vi "FTW-File-ResolveSymbolicPaths.vi"(0 "Unresolved Path":path, 11 "error in":errorcluster) -> (4 "Resolved Path":path, 15 "error out":errorcluster)   [LabVIEW 2012]
uses:
  Error/FTW-ERR-ThrowError.vi
panel:
  # "Inputs"
  # "Outputs"
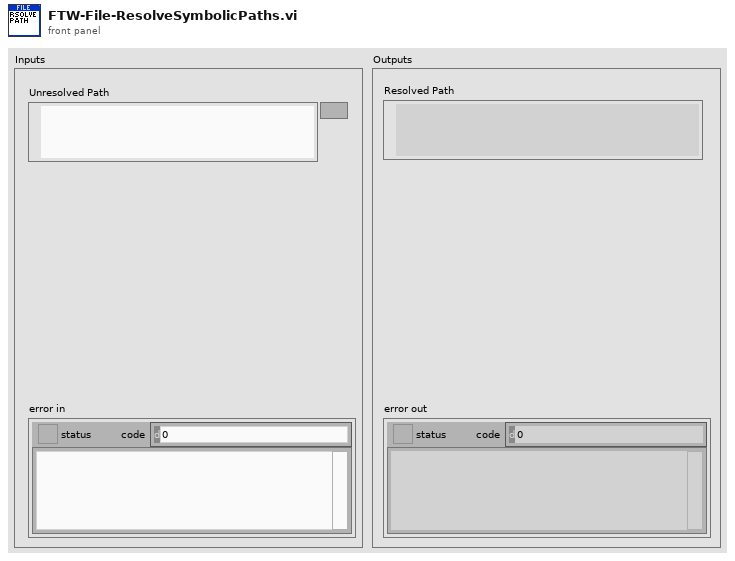
[diagram p1: front panel]
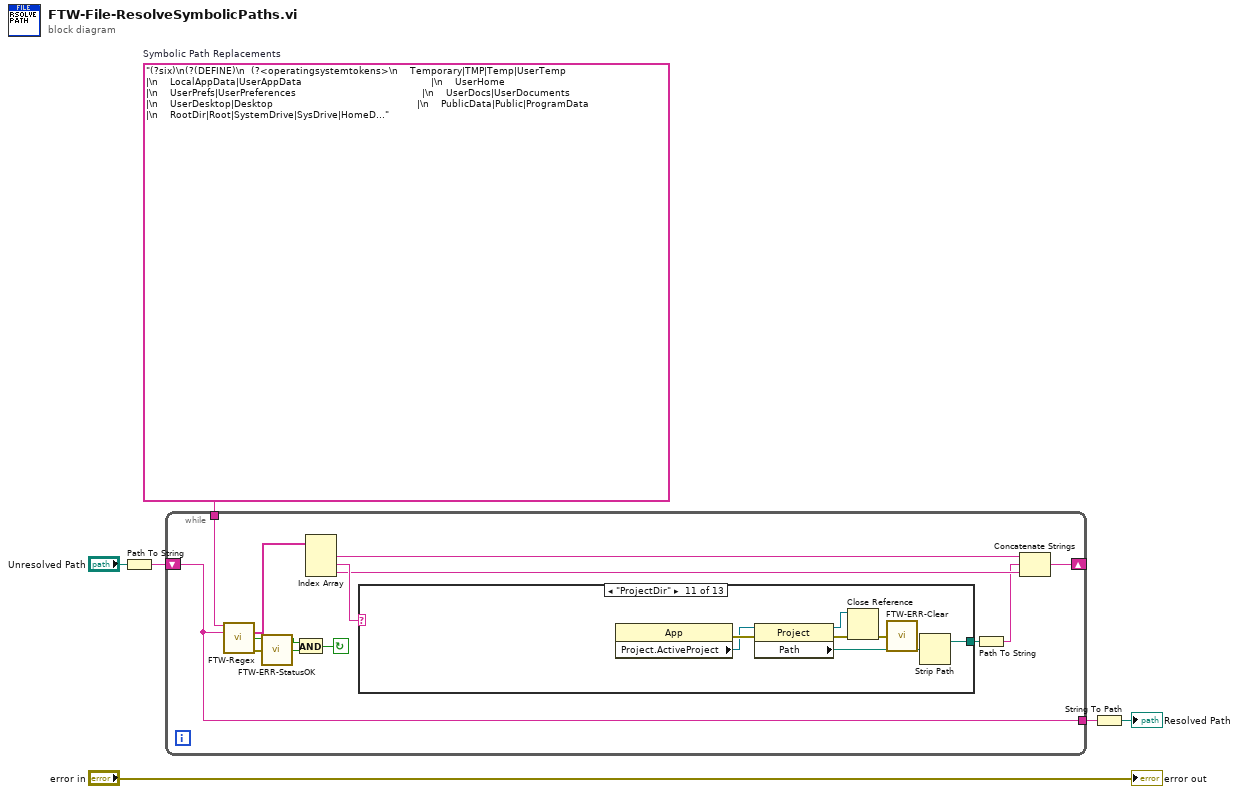
[diagram p0: block diagram]
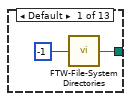
[diagram p2: hidden frame]
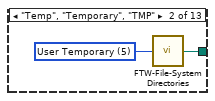
[diagram p3: hidden frame]
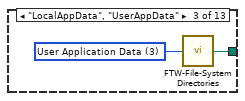
[diagram p4: hidden frame]
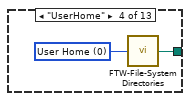
[diagram p5: hidden frame]
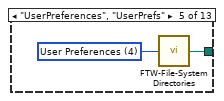
[diagram p6: hidden frame]
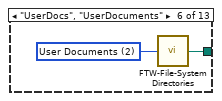
[diagram p7: hidden frame]
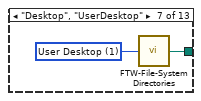
[diagram p8: hidden frame]
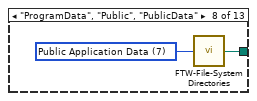
[diagram p9: hidden frame]
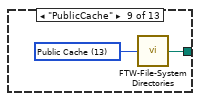
[diagram p10: hidden frame]
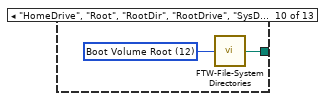
[diagram p11: hidden frame]
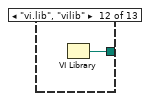
[diagram p12: hidden frame]
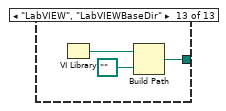
[diagram p13: hidden frame]
diagram:
  w3 = "(?six)\n(?(DEFINE)\n  (?<operatingsystemtokens>\n    Temporary|TMP|Temp|UserTemp                                        |\n    LocalAppData|UserAppData                                           |\n    UserHome                                                           |\n    UserPrefs|UserPreferences                                          |\n    UserDocs|UserDocuments                                             |\n    UserDesktop|Desktop                                                |\n    PublicData|Public|ProgramData                                      |\n    RootDir|Root|SystemDrive|SysDrive|HomeDrive|RootDrive|SystemRoot\n  )\n  (?<labviewdirectorytokens>\n    ### LabVIEW-specific Tokens ###\n    ProjectDir                        |\n    resource                          |\n    vilib|vi\\.lib                     |\n    LabVIEWBaseDir|LabVIEW\n  )\n)\n\n### Allow OS tokens to be between [], %%, or <>\n### Allow LabVIEW tokens to be between [] or <>\n### Each symbolic path has an optional trailing colon (:)\n(\\A.*?)\n(?: \\[(  (?&operatingsystemtokens)  |  (?&labviewdirectorytokens)  )\\]:? |\n    \\<(  (?&operatingsystemtokens)  |  (?&labviewdirectorytokens)  )\\>:? |\n    \\%(  (?&operatingsystemtokens)                                 )\\%:? )\n(.*?\\z)"  # Symbolic Path Replacements
  n1 = Path To String(path="Unresolved Path") -> (string=w1:string)
  n2 = while {
    tunnel: w3 -> [w15]
    tunnel: [w12] -> w2
    shift-right: [w11] -> _
    shift-left: w1 -> [w12]
    stop <- w16 continue-if-true
    n3 = call "FTW-Regex.vi"("Regular Expression"=w15, "Input String"=w12) -> ("Submatches"=w14:string[], "Match Found?"=w18:bool, "error out"=w19:errorcluster)  [unwired: 9 in, 2 out]
    n4 = call "FTW-ERR-StatusOK.vi"("error to check"=w19) -> ("Status OK?"=w17:bool)
    n5 = And(x=w18, y=w17) -> (x .and. y?=w16:bool)
    n6 = Index Array(array=w14) -> (element #1=w10:string, element #2=w13:string, element #3=w9:string)  [unwired: 3 in]
    n7 = case shown="\"ProjectDir\"" w13 {
      tunnel: [w20 w23 w25 w27 w29 w31 w33 w34 w36 w38 w40 w47 w49] -> w7
      frame Default {
        n8 = call "FTW-File-SystemDirectories.vi"("System Directory"=-1) -> ("Directory"=w20:path)
      }
      frame "Temp", "Temporary", "TMP" {
        w22 = 5 items=["User Home"=0, "User Desktop"=1, "User Documents"=2, "User Application Data"=3, "User Preferences"=4, "User Temporary"=5, "Public Documents"=6, "Public Application Data"=7, "Public Preferences"=8, "Public Cache"=13, "System Core Libraries"=9, "System Installed Libraries"=10, "Application Files"=11, "Boot Volume Root"=12] ("System Directory")
        n9 = call "FTW-File-SystemDirectories.vi"("System Directory"=w22) -> ("Directory"=w23:path)
      }
      frame "LocalAppData", "UserAppData" {
        w24 = 3 items=["User Home"=0, "User Desktop"=1, "User Documents"=2, "User Application Data"=3, "User Preferences"=4, "User Temporary"=5, "Public Documents"=6, "Public Application Data"=7, "Public Preferences"=8, "Public Cache"=13, "System Core Libraries"=9, "System Installed Libraries"=10, "Application Files"=11, "Boot Volume Root"=12] ("System Directory")
        n10 = call "FTW-File-SystemDirectories.vi"("System Directory"=w24) -> ("Directory"=w25:path)
      }
      frame "UserHome" {
        w26 = 0 items=["User Home"=0, "User Desktop"=1, "User Documents"=2, "User Application Data"=3, "User Preferences"=4, "User Temporary"=5, "Public Documents"=6, "Public Application Data"=7, "Public Preferences"=8, "Public Cache"=13, "System Core Libraries"=9, "System Installed Libraries"=10, "Application Files"=11, "Boot Volume Root"=12] ("System Directory")
        n11 = call "FTW-File-SystemDirectories.vi"("System Directory"=w26) -> ("Directory"=w27:path)
      }
      frame "UserPreferences", "UserPrefs" {
        w28 = 4 items=["User Home"=0, "User Desktop"=1, "User Documents"=2, "User Application Data"=3, "User Preferences"=4, "User Temporary"=5, "Public Documents"=6, "Public Application Data"=7, "Public Preferences"=8, "Public Cache"=13, "System Core Libraries"=9, "System Installed Libraries"=10, "Application Files"=11, "Boot Volume Root"=12] ("System Directory")
        n12 = call "FTW-File-SystemDirectories.vi"("System Directory"=w28) -> ("Directory"=w29:path)
      }
      frame "UserDocs", "UserDocuments" {
        w30 = 2 items=["User Home"=0, "User Desktop"=1, "User Documents"=2, "User Application Data"=3, "User Preferences"=4, "User Temporary"=5, "Public Documents"=6, "Public Application Data"=7, "Public Preferences"=8, "Public Cache"=13, "System Core Libraries"=9, "System Installed Libraries"=10, "Application Files"=11, "Boot Volume Root"=12] ("System Directory")
        n13 = call "FTW-File-SystemDirectories.vi"("System Directory"=w30) -> ("Directory"=w31:path)
      }
      frame "Desktop", "UserDesktop" {
        w32 = 1 items=["User Home"=0, "User Desktop"=1, "User Documents"=2, "User Application Data"=3, "User Preferences"=4, "User Temporary"=5, "Public Documents"=6, "Public Application Data"=7, "Public Preferences"=8, "Public Cache"=13, "System Core Libraries"=9, "System Installed Libraries"=10, "Application Files"=11, "Boot Volume Root"=12] ("System Directory")
        n14 = call "FTW-File-SystemDirectories.vi"("System Directory"=w32) -> ("Directory"=w33:path)
      }
      frame "ProgramData", "Public", "PublicData" {
        w35 = 7 items=["User Home"=0, "User Desktop"=1, "User Documents"=2, "User Application Data"=3, "User Preferences"=4, "User Temporary"=5, "Public Documents"=6, "Public Application Data"=7, "Public Preferences"=8, "Public Cache"=13, "System Core Libraries"=9, "System Installed Libraries"=10, "Application Files"=11, "Boot Volume Root"=12] ("System Directory")
        n15 = call "FTW-File-SystemDirectories.vi"("System Directory"=w35) -> ("Directory"=w34:path)
      }
      frame "PublicCache" {
        w37 = 13 items=["User Home"=0, "User Desktop"=1, "User Documents"=2, "User Application Data"=3, "User Preferences"=4, "User Temporary"=5, "Public Documents"=6, "Public Application Data"=7, "Public Preferences"=8, "Public Cache"=13, "System Core Libraries"=9, "System Installed Libraries"=10, "Application Files"=11, "Boot Volume Root"=12] ("System Directory")
        n16 = call "FTW-File-SystemDirectories.vi"("System Directory"=w37) -> ("Directory"=w36:path)
      }
      frame "HomeDrive", "Root", "RootDir", "RootDrive", "SysDrive", "SystemDrive", "SystemRoot" {
        w39 = 12 items=["User Home"=0, "User Desktop"=1, "User Documents"=2, "User Application Data"=3, "User Preferences"=4, "User Temporary"=5, "Public Documents"=6, "Public Application Data"=7, "Public Preferences"=8, "Public Cache"=13, "System Core Libraries"=9, "System Installed Libraries"=10, "Application Files"=11, "Boot Volume Root"=12] ("System Directory")
        n17 = call "FTW-File-SystemDirectories.vi"("System Directory"=w39) -> ("Directory"=w38:path)
      }
      frame "ProjectDir" {
        n18 = property class="App"() -> (error out=w43:errorcluster, "Project.ActiveProject"=w42:refnum<vi>)  [unwired: 2 in, 1 out]
        n19 = property class="Project"(reference=w42, error in=w43) -> (reference out=w44:refnum<vi>, error out=w45:errorcluster, "Path"=w41:path)
        n20 = Close Reference(reference=w44, error in (no error)=w45) -> (error out=w46:errorcluster)
        n21 = call "FTW-ERR-Clear.vi"("error to snuff"=w46) -> ()  [unwired: 1 out]
        n22 = Strip Path(path=w41) -> (stripped path=w40:path)  [unwired: 1 out]
      }
      frame "vi.lib", "vilib" {
        n23 = VI Library() -> (path=w47:path)
      }
      frame "LabVIEW", "LabVIEWBaseDir" {
        n24 = VI Library() -> (path=w50:path)
        n25 = Build Path(base path=w50, name or relative path=path ".." ("appended path")) -> (appended path=w49:path)
      }
    }
    n26 = Path To String(path=w7) -> (string=w8:string)
    n27 = Concatenate Strings(w10, w8, w9) -> (w11:string)
  }
  n28 = String To Path(string=w2) -> (path=→"Resolved Path":path)
  "error out" <- "error in"
